vi "Cumulative Moving Average (SubVI).vi"(9 "(n)":i32, 10 "CMA (n)":dbl, 11 "x (n+1)":dbl) -> (3 "CMA (n+1)":dbl)   [LabVIEW 2017]
panel:
  # "This simple subVI calculates the Cumulative Moving Average based on the formula derived on wikipedia.\nhttps://en.wikipedia.org/wiki/Moving_average#Cumulative_moving_average"
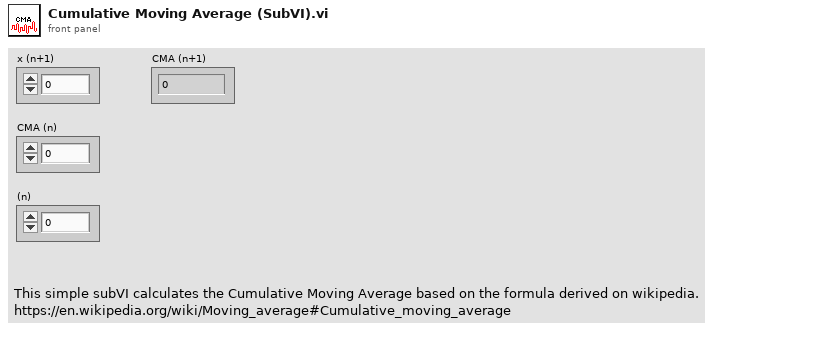
[diagram p1: front panel]
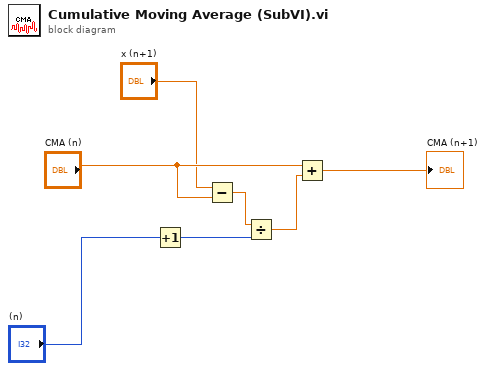
[diagram p0: block diagram]
diagram:
  n1 = Increment(x="(n)") -> (x+1=w7:i32)
  n2 = Subtract(x="x (n+1)", y="CMA (n)") -> (x-y=w3:dbl)
  n3 = Divide(x=w3, y=w7) -> (x/y=w4:dbl)
  n4 = Add(x="CMA (n)", y=w4) -> (x+y=→"CMA (n+1)":dbl)
